vi "Sign Mux.vi"(4 "Signed Number B":dbl, 5 "Unsigned Number A":dbl) -> (1 "Signed Number A":dbl)   [LabVIEW 2014]
uses:
  <vilib>/ptbypt/NI_PtbyPt.lvlib
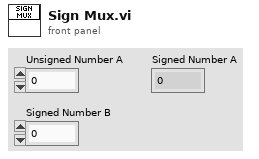
[diagram p1: front panel]
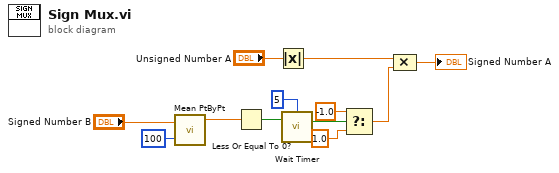
[diagram p0: block diagram]
diagram:
  n1 = call <vilib>:"Mean PtByPt.vi"("x"="Signed Number B", "sample length"=100) -> ("mean"=w2:dbl)  [unwired: 2 in, 1 out]
  n2 = Less Or Equal To 0?(x=w2) -> (x <= 0?=w9:bool)
  n3 = Absolute Value(x="Unsigned Number A") -> (abs(x)=w11:dbl)
  n4 = call "Wait Timer.vi"("Boolean In"=w9, "Timer"=u32 5) -> ("Boolean Out"=w7:bool)  [unwired: 3 in]
  n5 = Select(t=-1.0, s=w7, f=1.0) -> (s? t:f=w4:dbl)
  n6 = Compound Arithmetic op=MULTIPLY(w11, w4) -> (→"Signed Number A":dbl)
